vi "Write RIO interface.vi"(8 "error in":errorcluster, 10 "RIO interface":string="RIO0", 11 "Profibus Module configuration in":refnum<class "Profibus Module configuration.lvclass">) -> (0 "error out":errorcluster, 3 "Profibus Module configuration out":refnum<class "Profibus Module configuration.lvclass">)   [LabVIEW 2013, in "Profibus Module configuration.lvclass"]
uses:
  Profibus Module configuration.lvclass
  Profibus Module configuration.lvclass/Profibus Module configuration.ctl
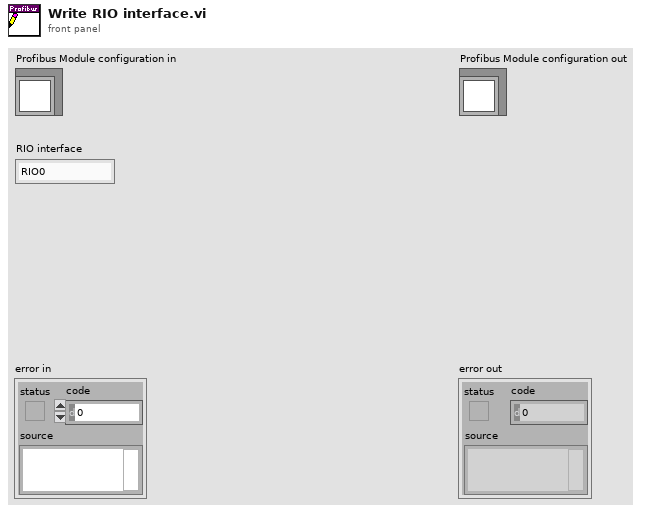
[diagram p1: front panel]
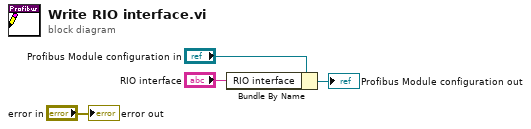
[diagram p0: block diagram]
diagram:
  n1 = Bundle By Name(cluster="Profibus Module configuration in", "RIO interface"="RIO interface") -> (→"Profibus Module configuration out":refnum<class "Profibus Module configuration.lvclass">)
  "error out" <- "error in"
